vi "BrakeWhenStop.vi"(11 "Motor Input":dbl) -> ()   [LabVIEW 2016]
uses:
  <vilib>/Rock Robotics/WPI/ThirdParty/CanMotor/TalonSRX/WPI_CANTalonSRX_BrakeOverride.ctl
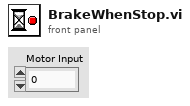
[diagram p1: front panel]
types:
  T1 = typedef "WPI_MotorControlDeviceRef.ctl" = cluster{"DeviceStatus":errorcluster, "Type":T2, "PWM":cluster{"PWM Channel":T3, "DeadBand":T4}, "CAN":cluster{"Device Number":u8, "SetOutput VI Ref":variant, "GetOutput VI Ref":variant, "Enable VI Ref":variant, "Disable VI Ref":variant, "Data":variant}, "Invert":bool}
  T2 = typedef "WPI_MotorControlType.ctl" = enum16{"PWM", "CAN"}
  T3 = typedef "FPGA_DIOPWMChannel.ctl" = enum8{"PWM 0", "PWM 1", "PWM 2", "PWM 3", "PWM 4", "PWM 5", "PWM 6", "PWM 7", "PWM 8", "PWM 9", "PWM MXP 0", "PWM MXP 1", "PWM MXP 2", "PWM MXP 3", "PWM MXP 4", "PWM MXP 5", "PWM MXP 6", "PWM MXP 7", "PWM MXP 8", "PWM MXP 9", "Invalid"}
  T4 = typedef "WPI_PWMDeadband.ctl" = cluster{"Name":string, "maxPositivePwm":i32, "minPositivePwm":i32, "centerPwm":i32, "maxNegativePwm":i32, "minNegativePwm":i32, "angularRange":u16}
  T5 = typedef "WPI_CANTalonSRX_BrakeOverride.ctl" = enum8{"No Override", "Override to Coast", "Override to Brake"}
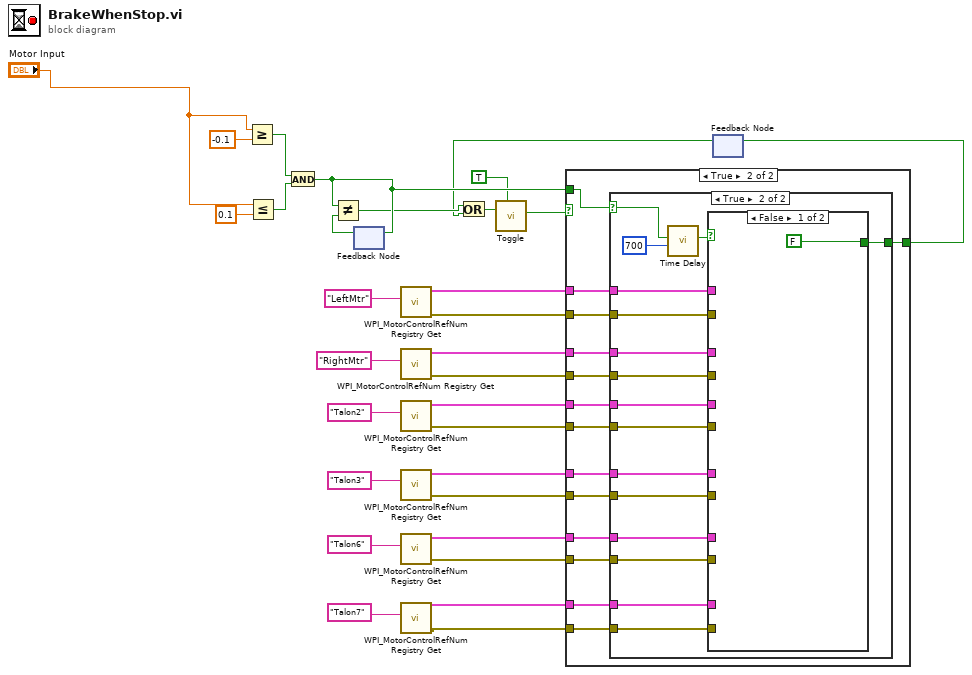
[diagram p0: block diagram]
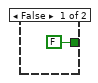
[diagram p2: hidden frame]
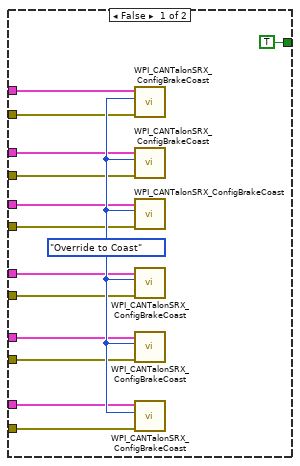
[diagram p3: hidden frame]
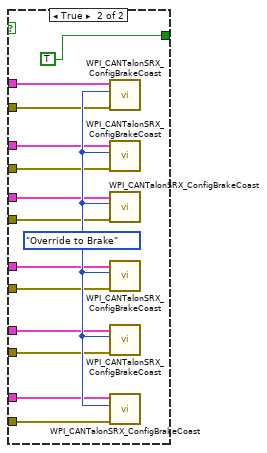
[diagram p4: hidden frame]
diagram:
  n1 = Greater Or Equal?(x="Motor Input", y=-0.1) -> (x >= y?=w29:bool)
  n2 = Less Or Equal?(x="Motor Input", y=0.1) -> (x <= y?=w30:bool)
  n3 = And(x=w29, y=w30) -> (x .and. y?=w26:bool)
  n4 = feedback #1() -> (w7:bool)  [unwired: 1 in]
  n5 = Not Equal?(x=w26, y=w7) -> (x != y?=w4:bool)
  n6 = feedback-in #1(w26) -> ()
  n7 = call <vilib>:"WPI_MotorControlRefNum Registry Get.vi"("refnum name"="LeftMtr") -> ("error out"=w14:errorcluster, "MotorControlDevRef"=w15:T1)  [unwired: 9 in]
  n8 = call <vilib>:"WPI_MotorControlRefNum Registry Get.vi"("refnum name"="RightMtr") -> ("error out"=w16:errorcluster, "MotorControlDevRef"=w17:T1)  [unwired: 9 in]
  n9 = call <vilib>:"WPI_MotorControlRefNum Registry Get.vi"("refnum name"="Talon2") -> ("error out"=w18:errorcluster, "MotorControlDevRef"=w19:T1)  [unwired: 9 in]
  n10 = call <vilib>:"WPI_MotorControlRefNum Registry Get.vi"("refnum name"="Talon3") -> ("error out"=w20:errorcluster, "MotorControlDevRef"=w21:T1)  [unwired: 9 in]
  n11 = call <vilib>:"WPI_MotorControlRefNum Registry Get.vi"("refnum name"="Talon6") -> ("error out"=w22:errorcluster, "MotorControlDevRef"=w23:T1)  [unwired: 9 in]
  n12 = call <vilib>:"WPI_MotorControlRefNum Registry Get.vi"("refnum name"="Talon7") -> ("error out"=w25:errorcluster, "MotorControlDevRef"=w24:T1)  [unwired: 9 in]
  n13 = feedback #2() -> (w2:bool)  [unwired: 1 in]
  n14 = Or(x=w4, y=w2) -> (x .or. y?=w5:bool)
  n15 = call "Toggle.vi"("Control"=TRUE, "Input"=w5) -> ("Output"=w6:bool)  [unwired: 9 in]
  n16 = case shown="True" w6 {
    tunnel: w26 -> [_ w46]
    tunnel: w14 -> [_ w45]
    tunnel: w15 -> [_ w44]
    tunnel: w16 -> [_ w43]
    tunnel: w17 -> [_ w42]
    tunnel: w18 -> [_ w41]
    tunnel: w19 -> [_ w40]
    tunnel: w20 -> [_ w39]
    tunnel: w21 -> [_ w38]
    tunnel: w22 -> [_ w37]
    tunnel: w23 -> [_ w36]
    tunnel: w24 -> [_ w35]
    tunnel: w25 -> [_ w34]
    tunnel: [FALSE w33] -> w3
    frame False {
    }
    frame True {
      n17 = case shown="True" w46 {
        selector: w46 -> [_ w74]
        tunnel: w45 -> [w53 w73]
        tunnel: w44 -> [w52 w72]
        tunnel: w43 -> [w55 w71]
        tunnel: w42 -> [w54 w70]
        tunnel: w41 -> [w57 w69]
        tunnel: w40 -> [w56 w68]
        tunnel: w39 -> [w59 w67]
        tunnel: w38 -> [w58 w66]
        tunnel: w37 -> [w51 w65]
        tunnel: w36 -> [w50 w64]
        tunnel: w35 -> [w49 w63]
        tunnel: w34 -> [w48 w62]
        tunnel: [TRUE w61] -> w33
        frame False {
          w60 = WPI_CANTalonSRX_BrakeOverride."Override to Coast" ("Brake / Coast Mode")
          n18 = call <vilib>:"WPI_CANTalonSRX_ConfigBrakeCoast.vi"("error in (no error)"=w53, "Brake / Coast Mode"=w60, "CAN Talon SRX Ref"=w52) -> ()  [unwired: 7 in, 2 out]
          n19 = call <vilib>:"WPI_CANTalonSRX_ConfigBrakeCoast.vi"("error in (no error)"=w55, "Brake / Coast Mode"=w60, "CAN Talon SRX Ref"=w54) -> ()  [unwired: 7 in, 2 out]
          n20 = call <vilib>:"WPI_CANTalonSRX_ConfigBrakeCoast.vi"("error in (no error)"=w57, "Brake / Coast Mode"=w60, "CAN Talon SRX Ref"=w56) -> ()  [unwired: 7 in, 2 out]
          n21 = call <vilib>:"WPI_CANTalonSRX_ConfigBrakeCoast.vi"("error in (no error)"=w59, "Brake / Coast Mode"=w60, "CAN Talon SRX Ref"=w58) -> ()  [unwired: 7 in, 2 out]
          n22 = call <vilib>:"WPI_CANTalonSRX_ConfigBrakeCoast.vi"("error in (no error)"=w51, "Brake / Coast Mode"=w60, "CAN Talon SRX Ref"=w50) -> ()  [unwired: 7 in, 2 out]
          n23 = call <vilib>:"WPI_CANTalonSRX_ConfigBrakeCoast.vi"("error in (no error)"=w48, "Brake / Coast Mode"=w60, "CAN Talon SRX Ref"=w49) -> ()  [unwired: 7 in, 2 out]
        }
        frame True {
          n24 = call "Time Delay.vi"("Time Delay"=u32 700, "Boolean in"=w74) -> ("Boolean out"=w75:bool)  [unwired: 9 in]
          n25 = case shown="False" w75 {
            tunnel: w73 -> [_ w90]
            tunnel: w72 -> [_ w89]
            tunnel: w71 -> [_ w88]
            tunnel: w70 -> [_ w87]
            tunnel: w69 -> [_ w86]
            tunnel: w68 -> [_ w85]
            tunnel: w67 -> [_ w84]
            tunnel: w66 -> [_ w83]
            tunnel: w65 -> [_ w82]
            tunnel: w64 -> [_ w81]
            tunnel: w63 -> [_ w80]
            tunnel: w62 -> [_ w79]
            tunnel: [FALSE TRUE] -> w61
            frame False {
            }
            frame True {
              w91 = WPI_CANTalonSRX_BrakeOverride."Override to Brake" ("Brake / Coast Mode")
              n26 = call <vilib>:"WPI_CANTalonSRX_ConfigBrakeCoast.vi"("error in (no error)"=w90, "Brake / Coast Mode"=w91, "CAN Talon SRX Ref"=w89) -> ()  [unwired: 7 in, 2 out]
              n27 = call <vilib>:"WPI_CANTalonSRX_ConfigBrakeCoast.vi"("error in (no error)"=w88, "Brake / Coast Mode"=w91, "CAN Talon SRX Ref"=w87) -> ()  [unwired: 7 in, 2 out]
              n28 = call <vilib>:"WPI_CANTalonSRX_ConfigBrakeCoast.vi"("error in (no error)"=w86, "Brake / Coast Mode"=w91, "CAN Talon SRX Ref"=w85) -> ()  [unwired: 7 in, 2 out]
              n29 = call <vilib>:"WPI_CANTalonSRX_ConfigBrakeCoast.vi"("error in (no error)"=w84, "Brake / Coast Mode"=w91, "CAN Talon SRX Ref"=w83) -> ()  [unwired: 7 in, 2 out]
              n30 = call <vilib>:"WPI_CANTalonSRX_ConfigBrakeCoast.vi"("error in (no error)"=w82, "Brake / Coast Mode"=w91, "CAN Talon SRX Ref"=w81) -> ()  [unwired: 7 in, 2 out]
              n31 = call <vilib>:"WPI_CANTalonSRX_ConfigBrakeCoast.vi"("error in (no error)"=w79, "Brake / Coast Mode"=w91, "CAN Talon SRX Ref"=w80) -> ()  [unwired: 7 in, 2 out]
            }
          }
        }
      }
    }
  }
  n32 = feedback-in #2(w3) -> ()
